vi "Axsun_GUI.vi"() -> ()   [LabVIEW 2018]
uses:
  Project/SerialSecOCT/SerialSectOCT/Software/Hardware Mfg/Axsun Laser/cluster_Axsun.ctl
  Action_Axsun.ctl
panel:
  out "output cluster":T1
  in  "stop":bool
  out "error out":errorcluster
  in  "Source Laser ON":bool
  in  "Laser OFF":bool
  in  "Source Laser OFF":bool
  in  "Laser On":bool
  # "double click to stop"
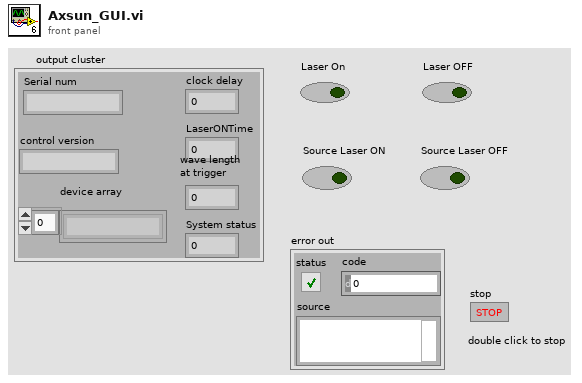
[diagram p1: front panel]
types:
  T1 = typedef "cluster_Axsun.ctl" = cluster{"device array":string[], "control version":string, "Serial num":string, "LaserONTime":i32, "wave length\nat trigger":dbl, "System status":dbl, "clock delay":u32}
  T2 = typedef "Action_Axsun.ctl" = enum16{"Init", "Stop", "Source current ON", "Source current OFF", "Laser ON", "Laser OFF", "GetLaserOnTime", "Clock delay"}
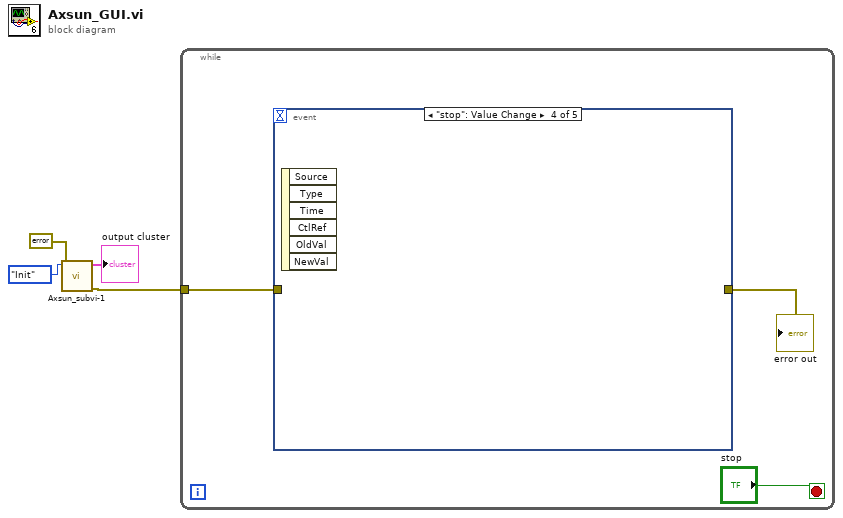
[diagram p0: block diagram]
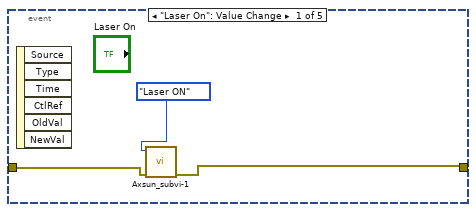
[diagram p2: hidden frame]
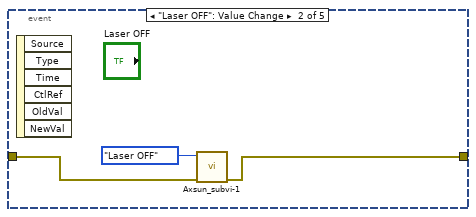
[diagram p3: hidden frame]
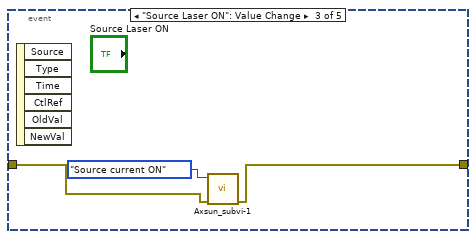
[diagram p4: hidden frame]
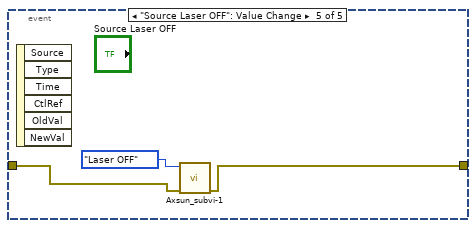
[diagram p5: hidden frame]
diagram:
  n1 = call "Axsun_subvi-1.vi"("error in (no error)"=errorcluster {"status"=FALSE, "code"=0, "source"=""}, "Action"=Action_Axsun."Init") -> ("error out"=w3:errorcluster, "output cluster"=→"output cluster":T1)  [unwired: 8 in]
  n2 = while {
    tunnel: w3 -> [w7]
    stop <- "stop" stop-if-true
    n3 = event shown="[3] \"stop\": Value Change" {
      selector: _ -> [_ _ _ _ _]
      dyn-events: _ -> [_ _ _ _ _]
      timeout: _ -> [_ _ _ _ _]
      tunnel: [w8 w11 w14 _ w17] -> w6
      tunnel: w7 -> [w9 w12 w16 _ w18]
      event "Laser On": Value Change {
        n4 = event-data() -> ()  [unwired: 1 in, 6 out]
        n5 = call "Axsun_subvi-1.vi"("error in (no error)"=w9, "Action"=Action_Axsun."Laser ON") -> ("error out"=w8:errorcluster)  [unwired: 8 in, 1 out]
      }
      event "Laser OFF": Value Change {
        n6 = event-data() -> ()  [unwired: 1 in, 6 out]
        n7 = call "Axsun_subvi-1.vi"("error in (no error)"=w12, "Action"=Action_Axsun."Laser OFF") -> ("error out"=w11:errorcluster)  [unwired: 8 in, 1 out]
      }
      event "Source Laser ON": Value Change {
        n8 = event-data() -> ()  [unwired: 1 in, 6 out]
        n9 = call "Axsun_subvi-1.vi"("error in (no error)"=w16, "Action"=Action_Axsun."Source current ON") -> ("error out"=w14:errorcluster)  [unwired: 8 in, 1 out]
      }
      event "stop": Value Change {
        n10 = event-data() -> ()  [unwired: 1 in, 6 out]
      }
      event "Source Laser OFF": Value Change {
        n11 = event-data() -> ()  [unwired: 1 in, 6 out]
        n12 = call "Axsun_subvi-1.vi"("error in (no error)"=w18, "Action"=Action_Axsun."Laser OFF") -> ("error out"=w17:errorcluster)  [unwired: 8 in, 1 out]
      }
    }
    "error out" <- w6
  }
